vi "Read From Driver.vi"(0 "error in":errorcluster, 1 "task in":refnum<k21>) -> (2 "error out":errorcluster, 3 "data":dbl[](array[numeric]), 4 "task out":refnum<k21>)   [LabVIEW 2011, in "PXIe-433x Custom Device.lvlib"]
uses:
  PXIe-433x Custom Device.lvlib
  <vilib>/DAQmx/read.llb/DAQmx Read (Analog 2D DBL NChan NSamp).vi
  <vilib>/DAQmx/miscellaneous.llb/DAQmx Fill In Error Info.vi
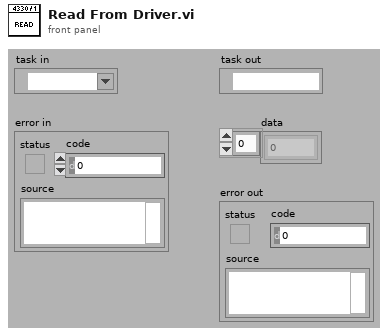
[diagram p1: front panel]
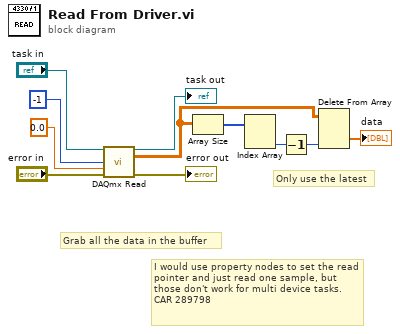
[diagram p0: block diagram]
diagram:
  # "I would use property nodes to set the read pointer and just read one sample, but those don't work for multi device tasks. CAR 289798"
  # "Only use the latest"
  # "Grab all the data in the buffer"
  n1 = call-poly <vilib>:"DAQmx Read.vi"("task/channels in"="task in", "number of samples per channel"=-1, "timeout"=0.0, "error in"="error in") -> ("task out"=→"task out":refnum<k21>, "data"=w4:dbl[][], "error out"=→"error out":errorcluster)  [unwired: 9 in]
  n2 = Array Size(array=w4) -> (size(s)=w3:i32[])
  n3 = Index Array(array=w3) -> (element #2=w2:i32)  [unwired: 2 in, 1 out]
  n4 = Decrement(x=w2) -> (x-1=w1:i32)
  n5 = Delete From Array(array=w4, index (col)=w1) -> (deleted portion=→"data":dbl[])  [unwired: 2 in, 1 out]
